vi "Channels.Inline.Write.Channel Pointer.vi"(8 "error in (no error)":errorcluster, 10 "Value in":dbl, 11 "Channel Pointer":u64) -> (0 "error out":errorcluster, 2 "Value out":dbl, 3 "Channel Pointer dup":u64)   [LabVIEW 2016, in "VeriStand Data.lvlib"]
uses:
  VeriStand Data.lvlib
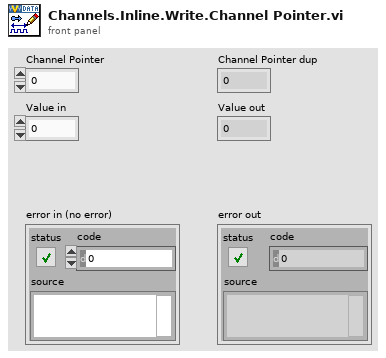
[diagram p1: front panel]
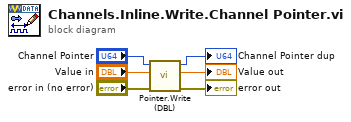
[diagram p0: block diagram]
diagram:
  n1 = call "Pointer.Write (DBL).vi"("error in (no error)"="error in (no error)", "value"="Value in", "pointer in"="Channel Pointer") -> ("error out"=→"error out":errorcluster, "value out"=→"Value out":dbl, "pointer out"=→"Channel Pointer dup":u64)  [unwired: 6 in]
